vi "Read Frame (ARGB Next).vi"(8 "error in (no error)":errorcluster, 10 "ARGB Image in":T1, 11 "Reader in":refnum<class "Reader.lvclass">) -> (0 "error out":errorcluster, 2 "ARGB Image":T1, 3 "Reader":refnum<class "Reader.lvclass">)   [LabVIEW 2020, in "video_io.lvlib" / "Reader.lvclass"]
uses:
  Reader.lvclass
  image/ARGB Image.ctl
  Reader.lvclass/Reader.ctl
  Reader Frame Action.ctl
  9eeb12df-7581-4bcd-a397-18dbd97d2298.vi
  <vilib>/Utility/error.llb/Error Cluster From Error Code.vi
  image/image.lvlib
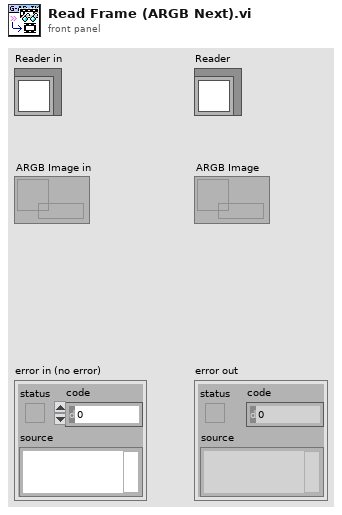
[diagram p1: front panel]
types:
  T1 = typedef "image.lvlib/ARGB Image.ctl" = refnum<data-value>
  T2 = typedef "video_io.lvlib/Reader.lvclass/Reader Frame Action.ctl" = enum8{"Frame at Index", "Frame at ms", "Next"}
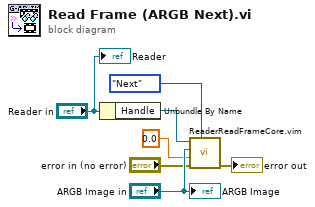
[diagram p0: block diagram]
diagram:
  n1 = Unbundle By Name("Reader in") -> ("Handle"=w6:refnum<data-value>)
  n2 = call "ReaderReadFrameCore.vim"("Reader Frame Action"=Reader_Frame_Action."Next", "error in (no error)"="error in (no error)", "Position"=0.0, "Greyscale Image"="ARGB Image in", "Handle"=w6) -> ("error out"=→"error out":errorcluster)  [unwired: 6 in]
  "Reader" <- "Reader in"
  "ARGB Image" <- "ARGB Image in"
